vi "whileLoop.vi"() -> ()   [LabVIEW 2015]
panel:
  in  "Button to stop":bool
  out "count":i32
  in  "Delay":dbl=1000.0
  out "LED":bool
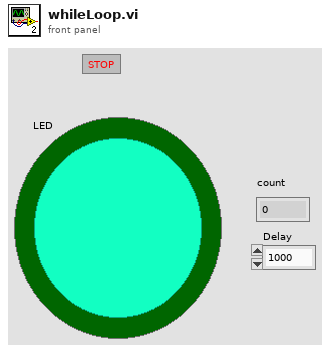
[diagram p1: front panel]
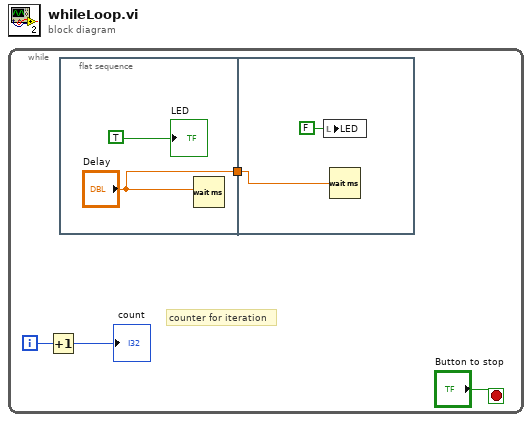
[diagram p0: block diagram]
diagram:
  n1 = while {
    i -> [w3]
    stop <- "Button to stop" stop-if-true
    # "counter for iteration"
    n2 = Increment(x=w3) -> (x+1=→"count":i32)
    n3 = flat-sequence {
      tunnel: ["Delay"] -> w4
      tunnel: w4 -> [w7]
      frame #0 {
        n4 = Wait (ms)(milliseconds to wait="Delay") -> ()  [unwired: 1 out]
        "LED" <- TRUE
      }
      frame #1 {
        n5 = local write "LED"(FALSE ("LED")) -> ()
        n6 = Wait (ms)(milliseconds to wait=w7) -> ()  [unwired: 1 out]
      }
    }
  }
